vi "Null Broadcast Events--constant.vi"() -> (3 "Sequence Engine Broadcast Events":T1)   [LabVIEW 2021, in "Sequence Engine.lvlib"]
doc: "Returns the broadcast events cluster with null references for defining the event types in a Register For Events function.\n_____\nBased on DQMH Dev Tools: Project Template 7.1.1.1528."
uses:
  Sequence Engine.lvlib
  Broadcast Events--cluster.ctl
  Did Init Argument--cluster.ctl
  Status Updated Argument--cluster.ctl
  Error Reported Argument--cluster.ctl
  Stop Argument--cluster.ctl
  Get Module Execution Status Argument--cluster.ctl
  New Test Result Argument--cluster.ctl
  Classes/Test Result/Result Data.ctl
  Classes/Test Result/Test Status.ctl
  Testing Started Argument--cluster.ctl
  Testing Completed Argument--cluster.ctl
  Retried Count Argument--cluster.ctl
  Classes/Test Result/Test Result.lvclass
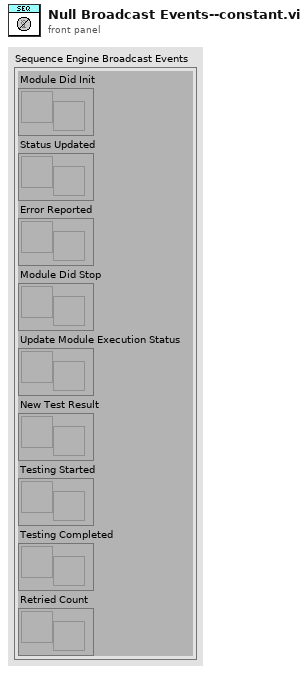
[diagram p1: front panel]
types:
  T1 = typedef "Sequence Engine.lvlib/Broadcast Events--cluster.ctl" = cluster{"Module Did Init":refnum<user-event>, "Status Updated":refnum<user-event>, "Error Reported":refnum<user-event>, "Module Did Stop":refnum<user-event>, "Update Module Execution Status":refnum<user-event>, "New Test Result":refnum<user-event>, "Testing Started":refnum<user-event>, "Testing Completed":refnum<user-event>, "Retried Count":refnum<user-event>}
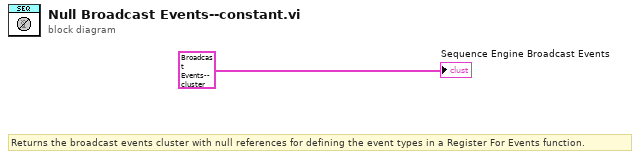
[diagram p0: block diagram]
diagram:
  # "Returns the broadcast events cluster with null references for defining the event types in a Register For Events function."
  "Sequence Engine Broadcast Events" <- T1 {"Module Did Init"=refnum, "Status Updated"=refnum, "Error Reported"=refnum, "Module Did Stop"=refnum, "Update Module Execution Status"=refnum, "New Test Result"=refnum, "Testing Started"=refnum, "Testing Completed"=refnum, "Retried Count"=refnum} ("Broadcast Events")
